vi "SetChSettings.vi"(0 "object in":refnum<class "AD2_DO_SDK.lvclass">, 2 "?":T1={"DO Trigger"={"secRun(0=Cont)"=0.0, "secWait"=0.0, "cRepeat(0=inf)"=0, "Repeat Trigger"=FALSE, "TrigrSrc"=enum."trigrsrcNone"}, "DO Ch Settings"=[{"Ch Index"=0, "Enable"=TRUE, "Clock DIvider"=500, "Type"=0, "DigitalOutOutput"=0, "IdleState"=0, "CounterData"={"NoHighBits"=20, "NoLowBits"=180, "NoInitialBits"=50, "Start High"=FALSE}, "Custom Data"={"countOfBits"=0, "rgBits"=[]}}, {"Ch Index"=1, "Enable"=TRUE, "Clock DIvider"=1000, "Type"=0, "DigitalOutOutput"=0, "IdleState"=0, "CounterData"={"NoHighBits"=100, "NoLowBits"=100, "NoInitialBits"=0, "Start High"=FALSE}, "Custom Data"={"countOfBits"=0, "rgBits"=[]}}]} {"DO Ch Settings"."IdleState" items=["PushPull", "OpenDrain", "OpenSource", "TriState"]; "DO Ch Settings"."DigitalOutOutput" items=["Pulse", "Custom", "Random"]; "DO Ch Settings"."Type" items=["Pulse", "Custom", "Random"]}, 5 "error in (no error)":errorcluster) -> (14 "object out":refnum<class "AD2_DO_SDK.lvclass">, 19 "error out":errorcluster)   [LabVIEW 2019, in "AD2_DO_SDK.lvclass"]
uses:
  AD2_DO_SDK.lvclass
  DOConfigurationData.ctl
  DOTrigger.ctl
  AD2_WFG_SDK_class/AD2TriggerSources.ctl
  DOSingleCh.ctl
  AD2_DO_SDK.lvclass/AD2_DO_SDK.ctl
  AD2_SDK_class/AD2_SDK.lvclass
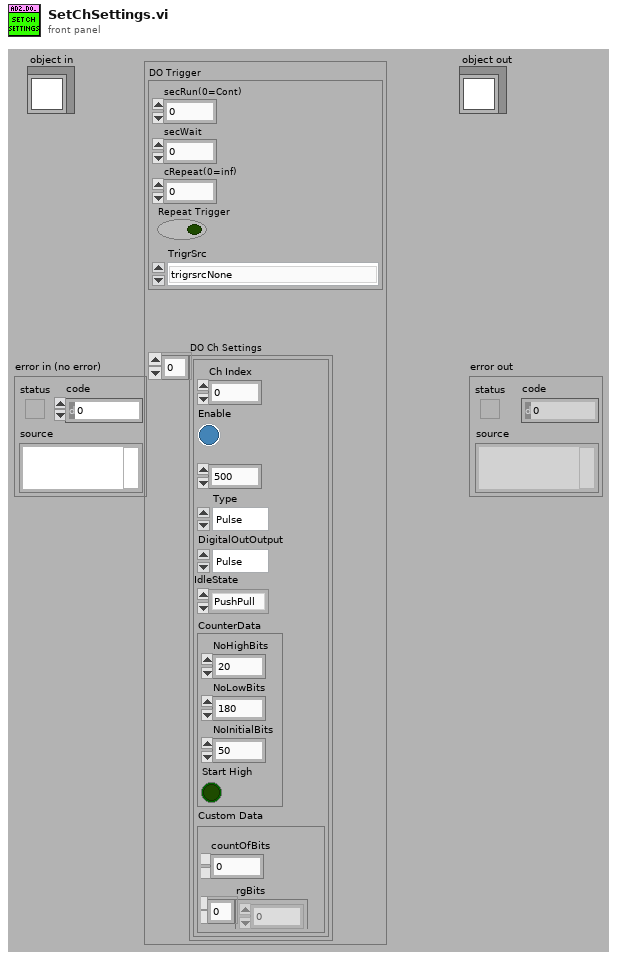
[diagram p1: front panel]
types:
  T1 = typedef "AD2_DO_SDK.lvclass/DOConfigurationData.ctl" = cluster{"DO Trigger":T2, "DO Ch Settings":T4[]}
  T2 = typedef "AD2_DO_SDK.lvclass/DOTrigger.ctl" = cluster{"secRun(0=Cont)":dbl, "secWait":dbl, "cRepeat(0=inf)":i32, "Repeat Trigger":bool, "TrigrSrc":T3}
  T3 = typedef "AD2_SDK.lvclass/AD2TriggerSources.ctl" = enum8{"trigrsrcNone", "trigsrcPC", "trigsrcDetectorAnalogIn", "trigsrcDetectorDigitalIn", "trigsrcAnalogIn", "trigsrcDigitalIn", "trigsrcDigitalOut", "trigsrcAnalogOut1", "trigsrcAnalogOut2", "trigsrcAnalogOut3", "trigsrcAnalogOut4", "trigsrcExternal1", "trigsrcExternal2", "trigsrcExternal3", "trigsrcExternal4", ""}
  T4 = typedef "AD2_DO_SDK.lvclass/DOSingleCh.ctl" = cluster{"Ch Index":i32, "Enable":bool, "Clock DIvider":u32, "Type":i32, "DigitalOutOutput":u16, "IdleState":u16, "CounterData":cluster{"NoHighBits":u32, "NoLowBits":u32, "NoInitialBits":u32, "Start High":bool}, "Custom Data":cluster{"countOfBits":u32, "rgBits":u8[]}}
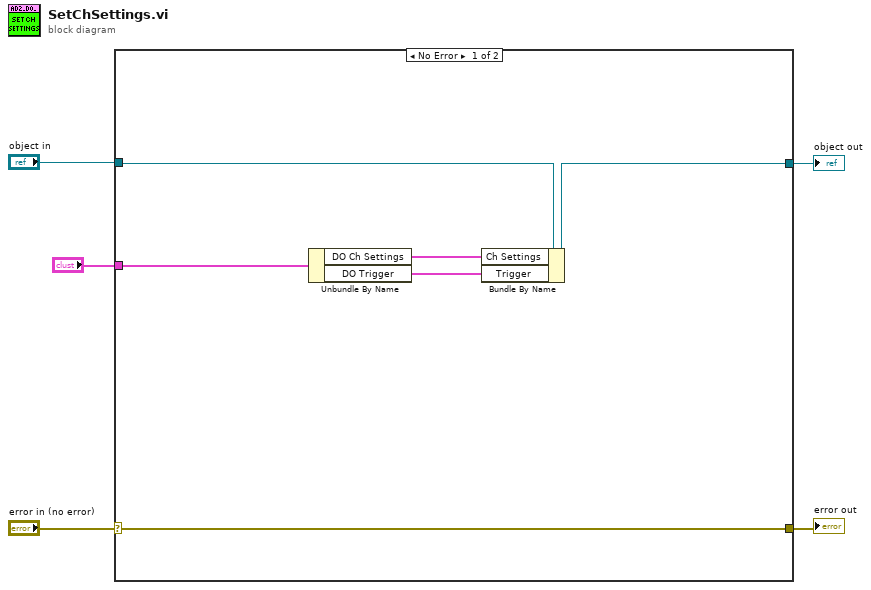
[diagram p0: block diagram]
diagram:
  n1 = case shown="No Error" "error in (no error)" {
    selector: "error in (no error)" -> [w11 w13]
    tunnel: [w11 w13] -> w4
    tunnel: [w9 w12] -> w2
    tunnel: "object in" -> [w10 w12]
    tunnel: "?" -> [w8 _]
    frame No Error {
      n2 = Unbundle By Name(w8) -> ("DO Ch Settings"=w7:T4[], "DO Trigger"=w6:T2)
      n3 = Bundle By Name(cluster=w10, "Ch Settings"=w7, "Trigger"=w6) -> (w9:refnum<class "AD2_DO_SDK.lvclass">)
    }
    frame Error {
    }
  }
  "error out" <- w4
  "object out" <- w2
